vi "Increment File Counter.vi"(8 "error in (no error)":errorcluster, 10 "File Path":path, 11 "Text File Sink in":refnum<class "Text File Sink.lvclass">) -> (0 "error out":errorcluster, 2 "File Path out":path, 3 "Text File Sink out":refnum<class "Text File Sink.lvclass">)   [LabVIEW 2017, in "Text File Sink.lvclass"]
uses:
  <vilib>/gpm_packages/@cs/event-logger/Source/Text File Sink/Text File Sink.lvclass
  <vilib>/gpm_packages/@cs/event-logger/Source/Text File Sink/Text File Sink.lvclass/Text File Sink.ctl
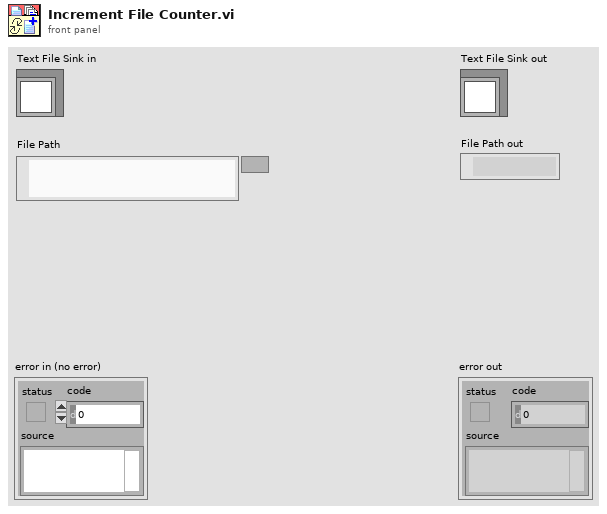
[diagram p1: front panel]
types:
  T1 = typedef "LVDateTimeRec.ctl" = cluster{"fractional second":dbl, "second":i32, "minute":i32, "hour":i32, "day of month":i32, "month":i32, "year":i32, "day of week":i32, "day of year":i32, "DST":i32}
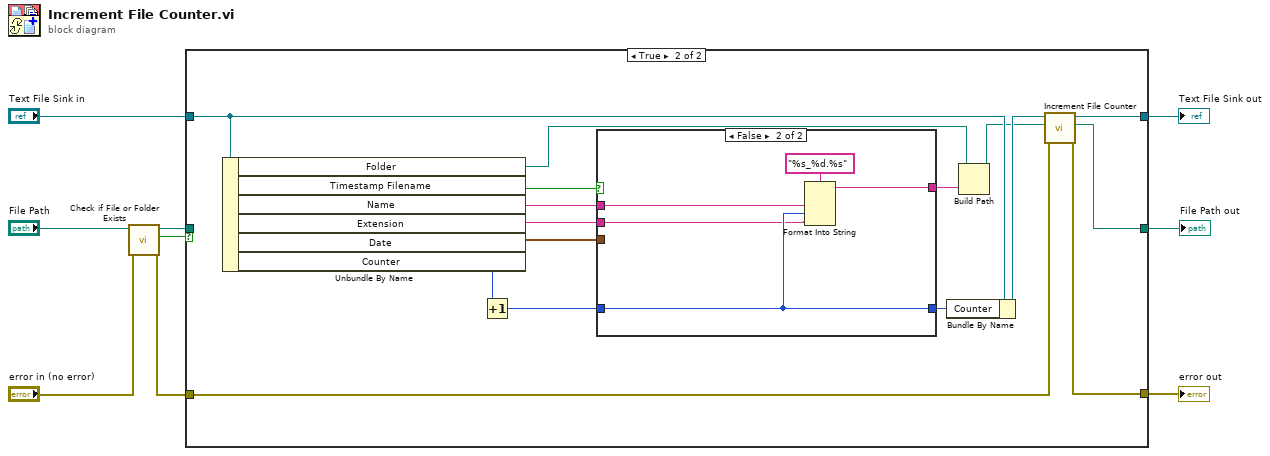
[diagram p0: block diagram]
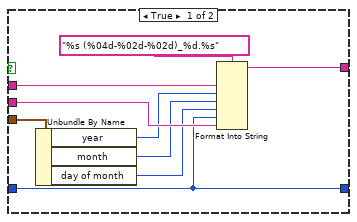
[diagram p3: hidden frame]
diagram:
  n1 = call <vilib>:"Check if File or Folder Exists.vi"("error in (no error)"="error in (no error)", "path"="File Path") -> ("error out"=w2:errorcluster, "file or folder exists?"=w9:bool, "dup path"=w8:path)  [unwired: 7 out]
  n2 = case shown="True" w9 {
    tunnel: w8 -> [w12 _]
    tunnel: [w12 w27] -> w3
    tunnel: [w11 w26] -> w6
    tunnel: "Text File Sink in" -> [w11 w28]
    tunnel: [w10 w24] -> w1
    tunnel: w2 -> [w10 w25]
    frame False {
    }
    frame True {
      n3 = Unbundle By Name(w28) -> ("Folder"=w19:path, "Timestamp Filename"=w13:bool, "Name"=w23:string, "Extension"=w22:string, "Date"=w21:T1, "Counter"=w17:u16)
      n4 = Increment(x=w17) -> (x+1=w18:u16)
      n5 = case shown="False" w13 {
        tunnel: w23 -> [w36 w41]
        tunnel: w22 -> [w35 w38]
        tunnel: w21 -> [w34 _]
        tunnel: [w30 w40] -> w20
        tunnel: w18 -> [w29 w39]
        tunnel: [w29 w39] -> w14
        frame True {
          n6 = Unbundle By Name(w34) -> ("year"=w33:i32, "month"=w32:i32, "day of month"=w31:i32)
          n7 = Format Into String(format string="%s (%04d-%02d-%02d)_%d.%s", w36, w33, w32, w31, w29, w35) -> (resulting string=w30:string)  [unwired: 2 in, 1 out]
        }
        frame False {
          n8 = Format Into String(format string="%s_%d.%s", w41, w39, w38) -> (resulting string=w40:string)  [unwired: 2 in, 1 out]
        }
      }
      n9 = Bundle By Name(cluster=w28, "Counter"=w14) -> (w16:refnum<class "Text File Sink.lvclass">)
      n10 = Build Path(base path=w19, name or relative path=w20) -> (appended path=w15:path)
      n11 = call <vilib>:"Increment File Counter.vi"("error in (no error)"=w25, "File Path"=w15, "Text File Sink in"=w16) -> ("error out"=w24:errorcluster, "File Path out"=w27:path, "Text File Sink out"=w26:refnum<class "Text File Sink.lvclass">)  [unwired: 6 in]
    }
  }
  "error out" <- w1
  "Text File Sink out" <- w6
  "File Path out" <- w3
